vi "converte_time_string_to_time_stamp.vi"(10 "input_string":string) -> (2 "date time rec":T1)   [LabVIEW 2020]
uses:
  <vilib>/Utility/miscctls.llb/LVDateTimeRec.ctl
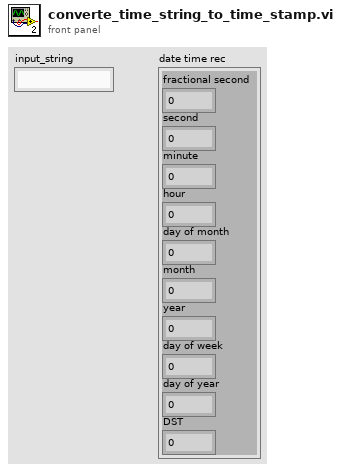
[diagram p1: front panel]
types:
  T1 = typedef "LVDateTimeRec.ctl" = cluster{"fractional second":dbl, "second":i32, "minute":i32, "hour":i32, "day of month":i32, "month":i32, "year":i32, "day of week":i32, "day of year":i32, "DST":i32}
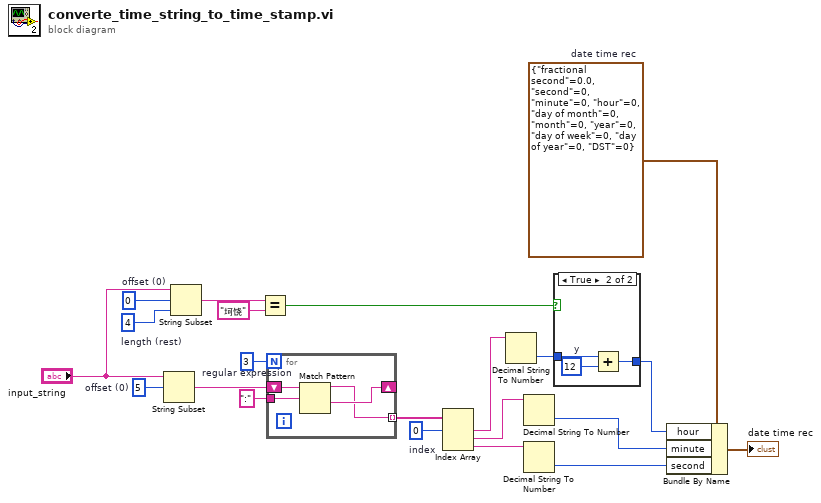
[diagram p0: block diagram]
diagram:
  w14 = 4  # length (rest)
  w13 = 0  # offset (0)
  w7 = 0  # index
  w4 = 5  # offset (0)
  w1 = ":"  # regular expression
  w2 = T1 {"fractional second"=0.0, "second"=0, "minute"=0, "hour"=0, "day of month"=0, "month"=0, "year"=0, "day of week"=0, "day of year"=0, "DST"=0}  # date time rec
  n1 = String Subset(string="input_string", offset (0)=w4) -> (substring=w5:string)  [unwired: 1 in]
  n2 = String Subset(string="input_string", offset (0)=w13, length (rest)=w14) -> (substring=w15:string)
  n3 = Equal?(x=w15, y="坷饶") -> (x = y?=w18:bool)
  n4 = for {
    N: 3 -> [_]
    shift-right: [w24] -> _
    shift-left: w5 -> [w25]
    tunnel: w1 -> [w23]
    tunnel: [w22] -> w12 mode=indexing
    n5 = Match Pattern(string=w25, regular expression=w23) -> (before substring=w22:string, after substring=w24:string)  [unwired: 1 in, 2 out]
  }
  n6 = Index Array "Index Array"(array=w12, index #1=w7) -> (element #1=w17:string, element #2=w8:string, element #3=w10:string)  [unwired: 2 in]
  n7 = Decimal String To Number(string=w17) -> (number=w19:i32)  [unwired: 2 in, 1 out]
  n8 = Decimal String To Number(string=w8) -> (number=w9:i32)  [unwired: 2 in, 1 out]
  n9 = Decimal String To Number(string=w10) -> (number=w11:i32)  [unwired: 2 in, 1 out]
  n10 = case shown="True" w18 {
    tunnel: w19 -> [w26 w29]
    tunnel: [w26 w27] -> w20
    frame False {
    }
    frame True {
      w28 = 12  # y
      n11 = Add(x=w29, y=w28) -> (x+y=w27:i32)
    }
  }
  n12 = Bundle By Name(cluster=w2, "hour"=w20, "minute"=w9, "second"=w11) -> (→"date time rec":T1)
